vi "data_inp(1).vi"() -> ()   [LabVIEW 2017]
uses:
  <instrlib>/Keithley 6517/Keithley 6517.lvlib
  <instrlib>/Lake Shore Cryotronics 332/Lake Shore Cryotronics 332.lvlib
panel:
  out "XY Graph":cluster{dbl[], dbl[]}(graph)
  out "appended array":dbl[][](array[numeric])
  in  "number of readings":i32
  out "Kelvin Reading":dbl min=0.0 max=1645.0 step=1e-05 format="%^.5e"
  in  "Lakeshore":refnum<visa-resource-name>
  out "Measurement 3":dbl
  in  "Keithley":refnum<visa-resource-name>
  out "Keithley_out":refnum<visa-resource-name>
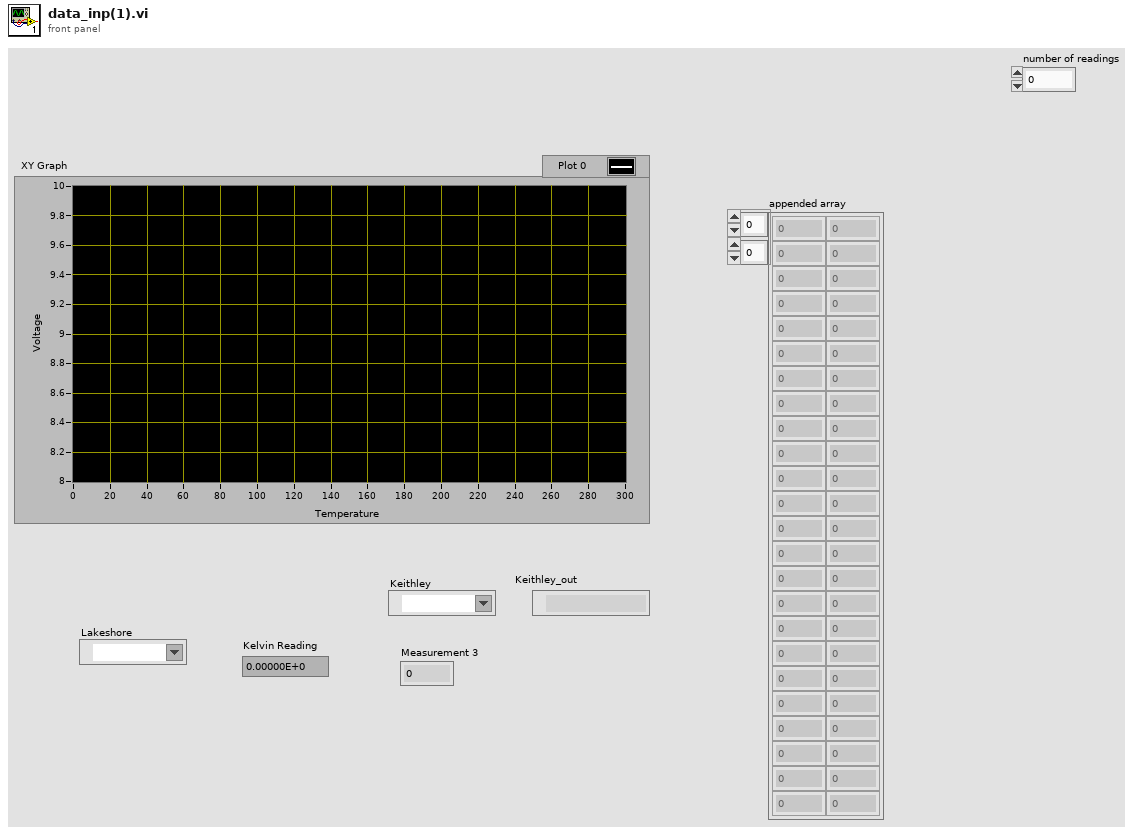
[diagram p1: front panel]
types:
  T1 = cluster{"Measurement":dbl, "Units":string, "Time Stamp and Date":string, "Reading #":dbl, "Channel #":dbl}
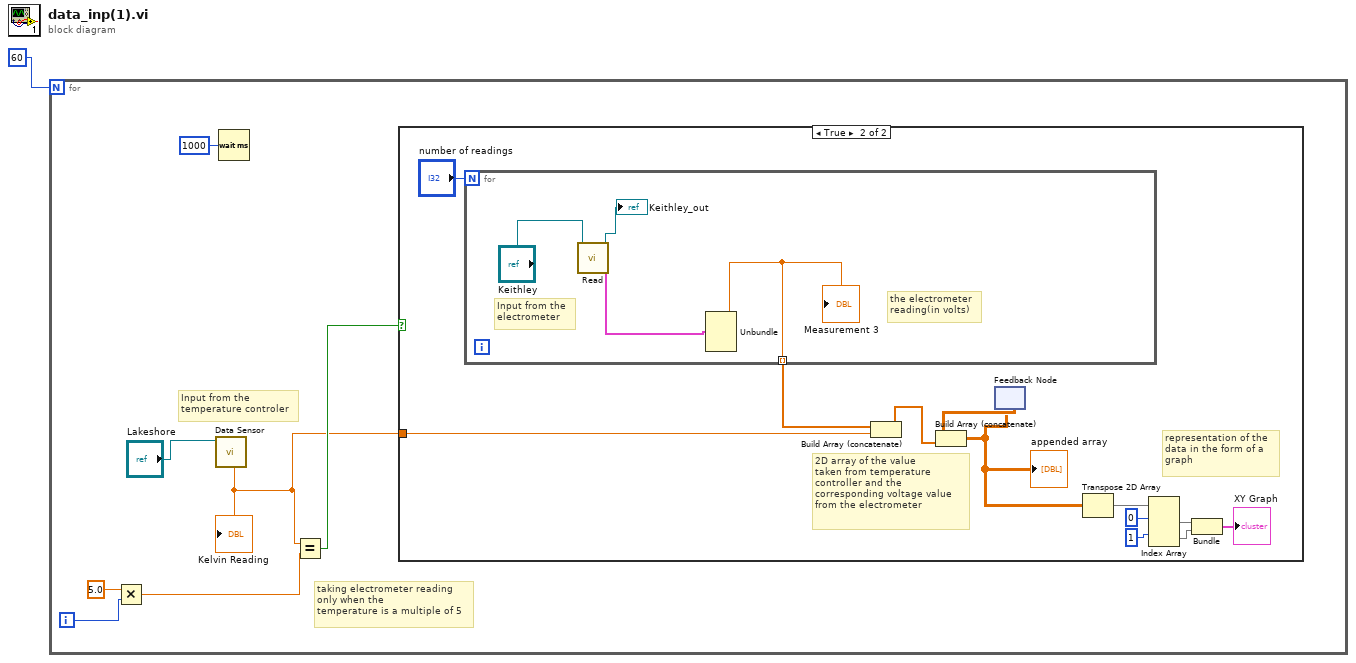
[diagram p0: block diagram]
diagram:
  n1 = for {
    N: 60 -> [_]
    i -> [w7]
    # "taking electrometer reading\nonly when the \ntemperature is a multiple of 5"
    # "Input from the \ntemperature controler"
    n2 = Multiply(x=5.0, y=w7) -> (x*y=w5:dbl)
    n3 = call <instrlib>:"Data Sensor.vi"("VISA resource name"="Lakeshore") -> ("Kelvin Reading"=w3:dbl)  [unwired: 6 in, 4 out]
    "Kelvin Reading" <- w3
    n4 = Wait (ms)(milliseconds to wait=u32 1000) -> ()  [unwired: 1 out]
    n5 = Equal?(x=w3, y=w5) -> (x = y?=w4:bool)
    n6 = case shown="True" w4 {
      tunnel: w3 -> [_ w9]
      frame False {
      }
      frame True {
        # "representation of the \ndata in the form of a\ngraph"
        # "2D array of the value\ntaken from temperature\ncontroller and the\ncorresponding voltage value \nfrom the electrometer"
        n7 = for {
          N: "number of readings" -> [_]
          tunnel: [w21] -> w10 mode=indexing
          # "the electrometer \nreading(in volts)"
          # "Input from the\nelectrometer"
          n8 = call <instrlib>:"Read.vi"("VISA resource name"="Keithley") -> ("Measurement"=w22:T1, "VISA resource name out"=→"Keithley_out":refnum<visa-resource-name>)  [unwired: 8 in, 1 out]
          n9 = Unbundle(w22) -> ("Measurement"=w21:dbl)  [unwired: 4 out]
          "Measurement 3" <- w21
        }
        n10 = Build Array (concatenate)(w10, w9) -> (w19:dbl[])
        n11 = feedback #1() -> (w18:dbl[][])  [unwired: 1 in]
        n12 = Build Array (concatenate)(w18, w19) -> (w11:dbl[][])
        "appended array" <- w11
        n13 = feedback-in #1(w11) -> ()
        n14 = Transpose 2D Array(2D array=w11) -> (transposed array=w12:dbl[][])
        n15 = Index Array(array=w12, index (row) #1=0 ("index (row)"), index (row) #2=1 ("index (row)")) -> (element #1=w15:dbl[], element #2=w14:dbl[])  [unwired: 2 in]
        n16 = Bundle(w15, w14) -> (→"XY Graph":cluster{dbl[], dbl[]})  [unwired: 1 in]
      }
    }
  }
